vi "IndividualSteering_f(x).vi"(3 "Error In":errorcluster, 4 "x":dbl) -> (0 "Error Out":errorcluster, 1 "y = f(x)":dbl)   [LabVIEW 2013]
uses:
  My Computer/Controls/IndividualSteering_f(x)_enum.ctl
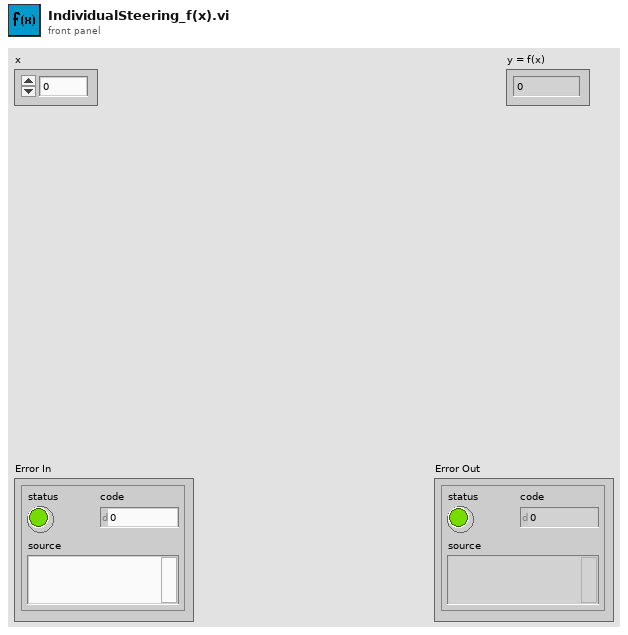
[diagram p1: front panel]
types:
  T1 = typedef "IndividualSteering_f(x)_enum.ctl" = enum16{"sin(x)", "cuttlefish sine", "cuttlefish triangle", "triangle"}
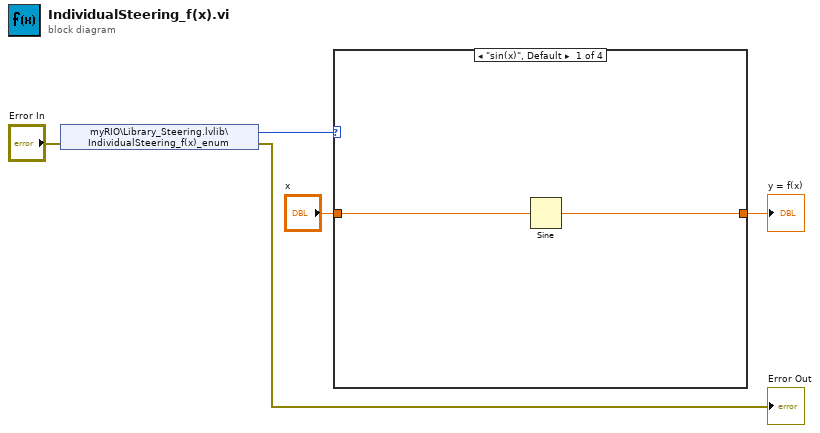
[diagram p0: block diagram]
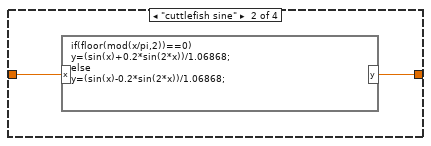
[diagram p2: hidden frame]
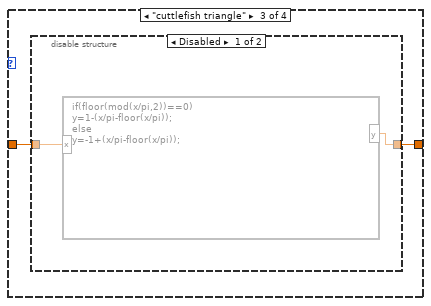
[diagram p3: hidden frame]
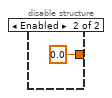
[diagram p4: hidden frame]
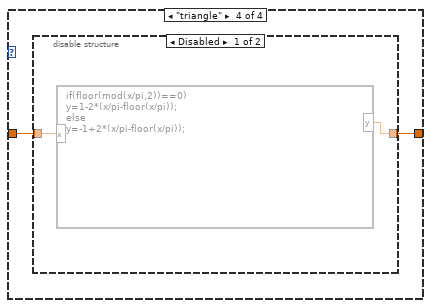
[diagram p5: hidden frame]
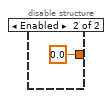
[diagram p6: hidden frame]
diagram:
  n1 = shared-variable "myRIO\\Library_Steering.lvlib\\IndividualSteering_f(x)_enum"(error in="Error In") -> (w3:T1, error out=→"Error Out":errorcluster)
  n2 = case shown="\"sin(x)\", Default" w3 {
    tunnel: "x" -> [w7 w9 w11 w16]
    tunnel: [w6 w8 w10 w15] -> w4
    frame "sin(x)", Default {
      n3 = Sine(x=w7) -> (sin(x)=w6:dbl)
    }
    frame "cuttlefish sine" {
      n4 = formula code="if(floor(mod(x/pi,2))==0)\ny=(sin(x)+0.2*sin(2*x))/1.06868;\nelse\ny=(sin(x)-0.2*sin(2*x))/1.06868;"("x"=w9) -> ("y"=w8:dbl)
    }
    frame "cuttlefish triangle" {
      n5 = disable-structure shown="Disabled" {
        disable-tunnel: w11 -> [w13 _]
        disable-tunnel: [w12 0.0 ("y")] -> w10
        frame Disabled {
          n6 = formula code="if(floor(mod(x/pi,2))==0)\ny=1-(x/pi-floor(x/pi));\nelse\ny=-1+(x/pi-floor(x/pi));"("x"=w13) -> ("y"=w12:dbl)
        }
        frame Enabled {
        }
      }
    }
    frame "triangle" {
      n7 = disable-structure shown="Disabled" {
        disable-tunnel: w16 -> [w18 _]
        disable-tunnel: [w17 0.0 ("y")] -> w15
        frame Disabled {
          n8 = formula code="if(floor(mod(x/pi,2))==0)\ny=1-2*(x/pi-floor(x/pi));\nelse\ny=-1+2*(x/pi-floor(x/pi));"("x"=w18) -> ("y"=w17:dbl)
        }
        frame Enabled {
        }
      }
    }
  }
  "y = f(x)" <- w4
